vi "Untitled 5.vi"() -> ()   [LabVIEW 2023]
panel:
  out "Particle Measurements (Pixels) (Particle Analysis 1)":dbl[][](array[numeric]) format="%.2f"
  out "Number of Particles (Particle Analysis 1)":i32
  in  "Stop (F)":bool
  out "Image Out":T1(plugin-control)
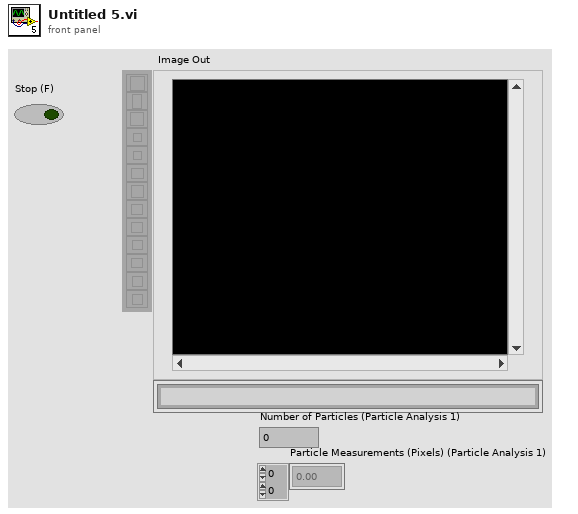
[diagram p1: front panel]
types:
  T1 = typedef "IMAQ Image.ctl" = refnum<image>
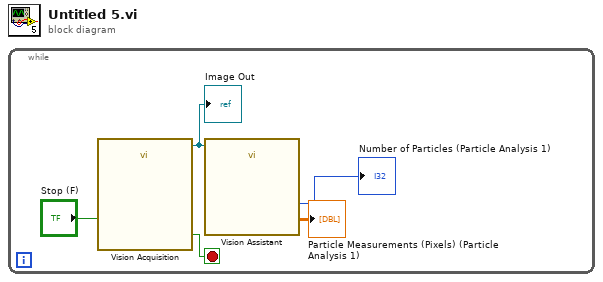
[diagram p0: block diagram]
diagram:
  n1 = while {
    stop <- w4 stop-if-true
    n2 = call "Vision Acquisition"("Stop (F)"="Stop (F)") -> ("Image Out"=w3:T1, "Stopped"=w4:bool)  [unwired: 24 in, 1 out]
    "Image Out" <- w3
    n3 = call "Vision Assistant"("Image In"=w3) -> ("Number of Particles (Particle Analysis 1)"=→"Number of Particles (Particle Analysis 1)":i32, "Particle Measurements (Pixels) (Particle Analysis 1)"=→"Particle Measurements (Pixels) (Particle Analysis 1)":dbl[][])  [unwired: 23 in, 2 out]
  }
